vi "main.vi"() -> ()   [LabVIEW 2023]
uses:
  #typedef_action.ctl
  #typedef_data.ctl
panel:
  in  "Massage":string="Error4025"
  out "String":string
  in  "Record max number":i32
  in  "Action":T1
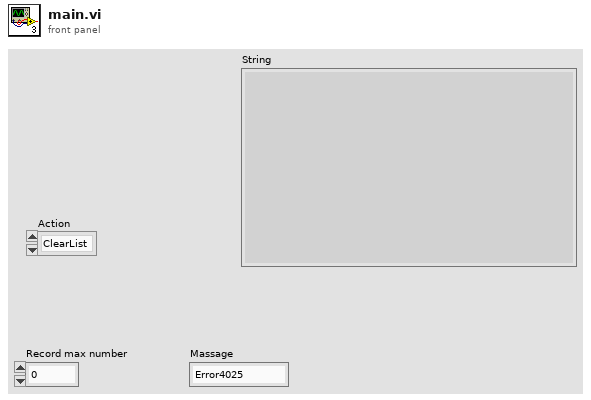
[diagram p1: front panel]
types:
  T1 = typedef "#typedef_action.ctl" = enum16{"ClearList", "AddRecord", "GetList"}
  T2 = typedef "#typedef_data.ctl" = cluster{"Date":timestamp, "Massage":string}
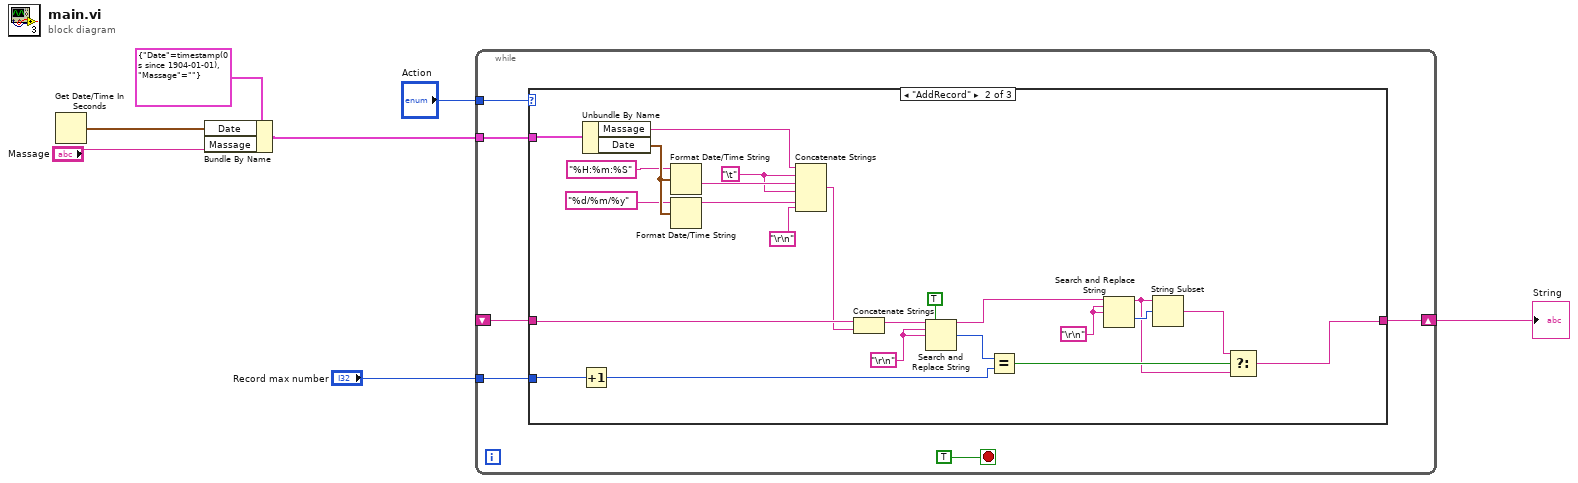
[diagram p0: block diagram]
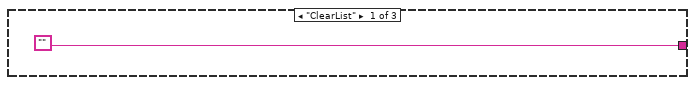
[diagram p2: hidden frame]
diagram:
  n1 = Get Date/Time In Seconds() -> (seconds since 1Jan1904=w4:timestamp)
  n2 = Bundle By Name(cluster=T2 {"Date"=timestamp(0 s since 1904-01-01), "Massage"=""} ("Data"), "Date"=w4, "Massage"="Massage") -> (w2:T2)
  n3 = while {
    tunnel: "Action" -> [w13]
    shift-right: [w12] -> w6
    shift-left: _ -> [w11]
    tunnel: w2 -> [w10]
    tunnel: "Record max number" -> [w8]
    stop <- TRUE stop-if-true
    n4 = case shown="\"AddRecord\"" w13 {
      tunnel: ["" w21 w39] -> w12
      tunnel: w11 -> [_ w29 w39]
      tunnel: w10 -> [_ w38 _]
      tunnel: w8 -> [_ w17 _]
      frame "ClearList" {
      }
      frame "AddRecord" {
        w19 = "\r\n"
        w20 = "\r\n"
        w31 = "\t"
        n5 = Increment(x=w17) -> (x+1=w16:i32)
        n6 = Unbundle By Name(w38) -> ("Massage"=w34:string, "Date"=w37:timestamp)
        n7 = Format Date/Time String(time format string (%c)="%H:%m:%S", seconds (now)=w37) -> (date/time string=w33:string)  [unwired: 1 in]
        n8 = Format Date/Time String(time format string (%c)="%d/%m/%y", seconds (now)=w37) -> (date/time string=w32:string)  [unwired: 1 in]
        n9 = Concatenate Strings(w34, w31, w33, w31, w32, "\r\n") -> (w28:string)
        n10 = Concatenate Strings(w29, w28) -> (w18:string)
        n11 = Search and Replace String(replace all?=TRUE ("replace all? (F)"), input string=w18, search string=w20, replace string=w20) -> (result string=w15:string, number of replacements=w26:i32)  [unwired: 4 in, 2 out]
        n12 = Equal?(x=w26, y=w16) -> (x = y?=w25:bool)
        n13 = Search and Replace String(input string=w15, search string=w19, replace string=w19) -> (result string=w23:string, offset past replacement=w24:i32)  [unwired: 5 in, 2 out]
        n14 = String Subset(string=w23, offset (0)=w24) -> (substring=w22:string)  [unwired: 1 in]
        n15 = Select(t=w22, s=w25, f=w23) -> (s? t:f=w21:string)
      }
      frame "GetList", Default {
      }
    }
  }
  "String" <- w6
